vi "server.vi"(8 "error in (no error)":errorcluster, 11 "RemoteAnalysisToolKit in":refnum<class "RemoteAnalysisToolKit.lvclass">) -> (0 "error out":errorcluster, 3 "RemoteAnalysisToolKit out":refnum<class "RemoteAnalysisToolKit.lvclass">)   [LabVIEW 2010, in "RemoteAnalysisToolKit.lvclass"]
uses:
  RemoteAnalysisToolKit.lvclass
  RemoteAnalysisToolKit.lvclass/RemoteAnalysisToolKit.ctl
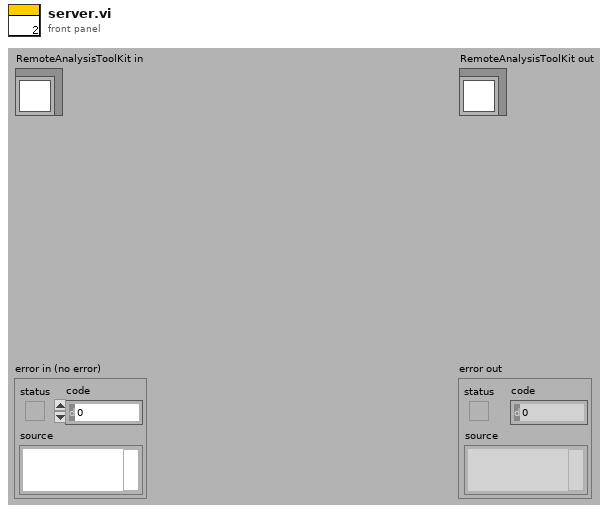
[diagram p1: front panel]
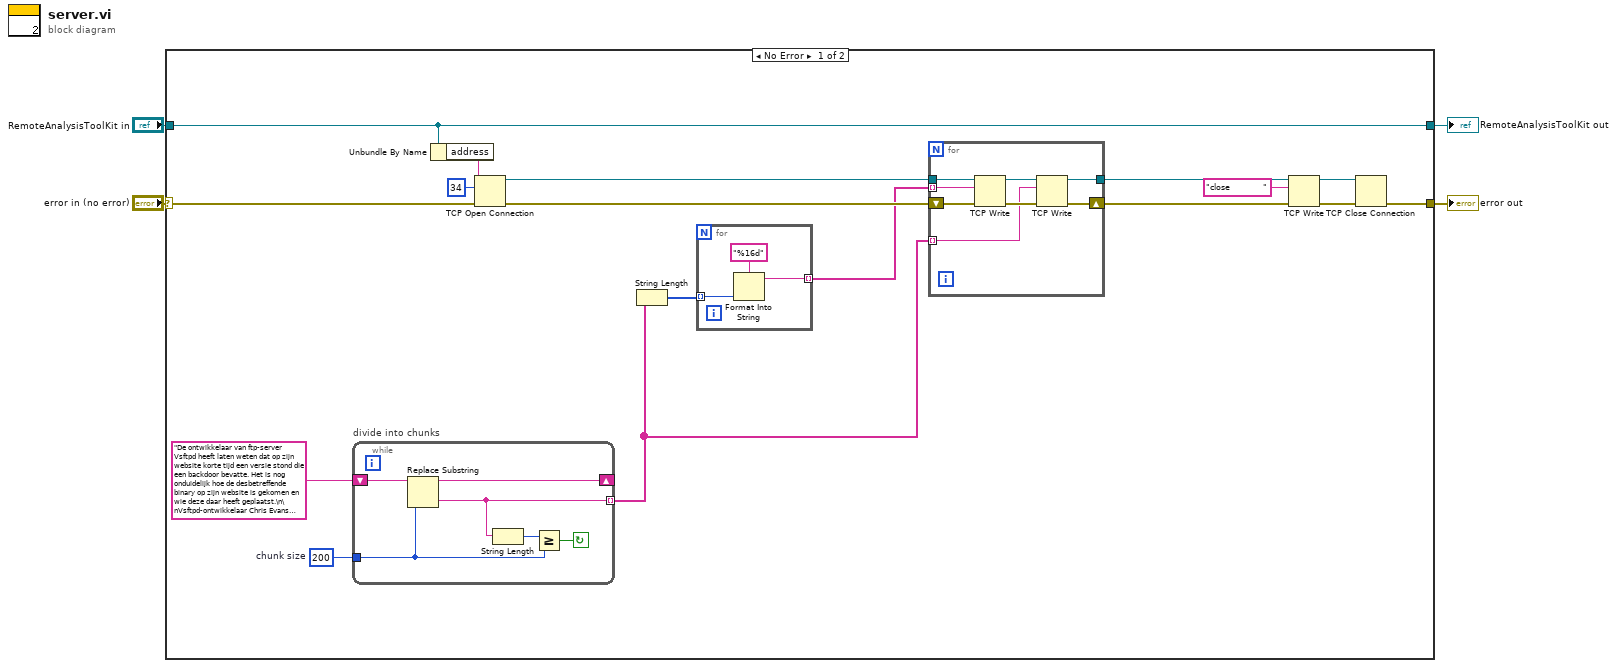
[diagram p0: block diagram]
diagram:
  n1 = case shown="No Error" "error in (no error)" {
    selector: "error in (no error)" -> [w6 w40]
    tunnel: [w5 w40] -> w3
    tunnel: [w20 w39] -> w2
    tunnel: "RemoteAnalysisToolKit in" -> [w20 w39]
    frame No Error {
      w16 = 200  # chunk size
      n2 = while "divide into chunks" {
        tunnel: [w35] -> w12 mode=indexing
        shift-right: [w36] -> _
        shift-left: "De ontwikkelaar van ftp-server Vsftpd heeft laten weten dat op zijn website korte tijd een versie stond die een backdoor bevatte. Het is nog onduidelijk hoe de desbetreffende binary op zijn website is gekomen en wie deze daar heeft geplaatst.\n\nVsftpd-ontwikkelaar Chris Evans schrijft op zijn blog dat hij een waarschuwing had ontvangen dat op de Vsftpd-site een tarball was aangetroffen die niet overeenkwam met de gpg-handtekening. Bij nader onderzoek bleek vsftpd-2.3.4.tar.gz, bedoeld voor Linux-systemen, een backdoor te bevatten. Een gebruiker die inlogt met gebruikersnaam ':)' op poort 6200, zou toegang krijgen tot een shell.\n\nHoe de gemanipuleerde Vsftpd-versie op de officiële website van de ftp-daemon is terechtgekomen, is onduidelijk. De software wordt door de ontwikkelaar gepromoot als zijnde 'zeer veilig'. Evans spreekt echter het vermoeden uit dat er kattenkwaad in het spel is; niet alleen wordt de backdoor nauwelijks verhuld, ook zou de ftp-daemon niet actief aan de buitenwereld kenbaar maken dat deze een achterdeur bevat. Desondanks heeft Evans besloten om zijn code voorlopig te hosten op Appspot." -> [w38]
        tunnel: w16 -> [w33]
        stop <- w37 continue-if-true
        n3 = Replace Substring(2:w33, 5:w38) -> (0:w35:string, 1:w36:string)  [unwired: 2 in]
        n4 = String Length(string=w35) -> (length=w34:i32)
        n5 = Greater Or Equal?(x=w34, y=w33) -> (x >= y?=w37:bool)
      }
      n6 = Unbundle By Name(w20) -> ("address"=w19:string)
      n7 = TCP Open Connection(address=w19, remote port or service name=u16 34, error in (no error)=w6) -> (connection ID=w18:refnum<k5>, error out=w17:errorcluster)  [unwired: 2 in]
      n8 = String Length(string=w12) -> (length=w14:i32[])
      n9 = for {
        tunnel: w14 -> [w31] mode=indexing
        tunnel: [w30] -> w13 mode=indexing
        n10 = Format Into String(format string="%16d", w31) -> (resulting string=w30:string)  [unwired: 2 in, 1 out]
      }
      n11 = for {
        tunnel: w18 -> [w29]
        tunnel: w13 -> [w25] mode=indexing
        tunnel: w12 -> [w24] mode=indexing
        tunnel: [w23] -> w11
        shift-right: [w22] -> w10
        shift-left: w17 -> [w28]
        n12 = TCP Write(connection ID=w29, data in=w25, error in (no error)=w28) -> (connection ID out=w26:refnum<k5>, error out=w27:errorcluster)  [unwired: 1 in, 1 out]
        n13 = TCP Write(connection ID=w26, data in=w24, error in (no error)=w27) -> (connection ID out=w23:refnum<k5>, error out=w22:errorcluster)  [unwired: 1 in, 1 out]
      }
      n14 = TCP Write(connection ID=w11, data in="close           ", error in (no error)=w10) -> (connection ID out=w8:refnum<k5>, error out=w7:errorcluster)  [unwired: 1 in, 1 out]
      n15 = TCP Close Connection(connection ID=w8, error in (no error)=w7) -> (error out=w5:errorcluster)  [unwired: 1 in, 1 out]
    }
    frame Error {
    }
  }
  "error out" <- w3
  "RemoteAnalysisToolKit out" <- w2
